vi "TestMain.vi"(11 "Array":string[](array[string])) -> (2 "source":string, 3 "code":i32)   [LabVIEW 2018]
panel:
  out "Failures":cluster{"Result":dbl, "Pass?":bool}[](array[cluster])
  in  "Test Points":dbl[][](array[numeric])
  out "error out":errorcluster
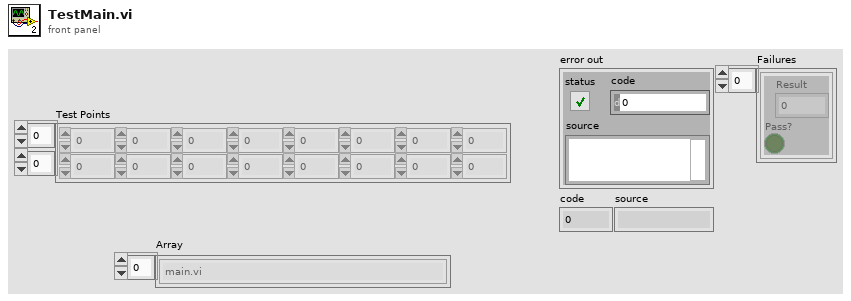
[diagram p1: front panel]
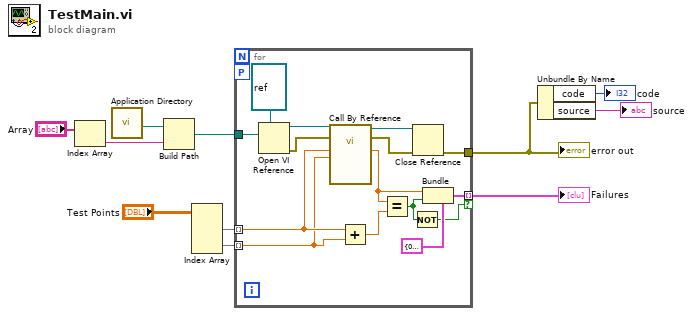
[diagram p0: block diagram]
diagram:
  n1 = Index Array(array="Array") -> (element=w4:string)  [unwired: 1 in]
  n2 = call <vilib>:"Application Directory.vi"() -> ("Application Directory"=w11:path)
  n3 = Build Path(base path=w11, name or relative path=w4) -> (appended path=w10:path)
  n4 = Index Array(array="Test Points") -> (element #1=w8:dbl[], element #2=w7:dbl[])  [unwired: 4 in]
  n5 = for {
    tunnel: w10 -> [w26]
    tunnel: [w21] -> w3
    tunnel: w8 -> [w19] mode=indexing
    tunnel: w7 -> [w18] mode=indexing
    workers-P: _ -> [_]
    tunnel: [w14] -> w6 mode=indexing if=w12
    n6 = Open VI Reference(type specifier VI Refnum (for type only)=refnum<vi> refnum, vi path=w26) -> (vi reference=w24:refnum<vi>, error out=w23:errorcluster)  [unwired: 4 in]
    n7 = call-by-ref "?"(reference=w24, error in=w23, "x"=w19, "y"=w18) -> (reference out=w20:refnum<vi>, error out=w22:errorcluster, "x+y"=w16:dbl)  [unwired: 13 in]
    n8 = Add(x=w19, y=w18) -> (x+y=w17:dbl)
    n9 = Equal?(x=w16, y=w17) -> (x = y?=w13:bool)
    n10 = Not(x=w13) -> (.not. x?=w12:bool)
    n11 = Close Reference(reference=w20, error in (no error)=w22) -> (error out=w21:errorcluster)
    n12 = Bundle(cluster=cluster{"Result":dbl, "Pass?":bool} {"Result"=0.0, "Pass?"=FALSE} ("Failures"), "Result"=w16, "Pass?"=w13) -> (w14:cluster{"Result":dbl, "Pass?":bool})
  }
  "error out" <- w3
  "Failures" <- w6
  n13 = Unbundle By Name(w3) -> ("code"=→"code":i32, "source"=→"source":string)
